vi "PROJE okuma dosya (1).vi"() -> ()   [LabVIEW 2017]
panel:
  out "Waveform Chart":i32[](graph)
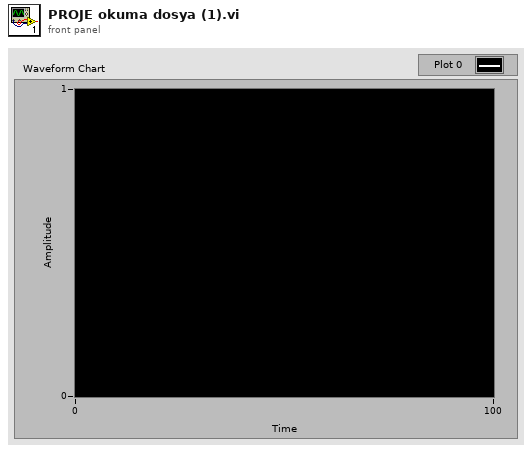
[diagram p1: front panel]
types:
  T1 = enum16{"open", "replace", "create", "open or create", "replace or create", "replace or create with confirmation"}
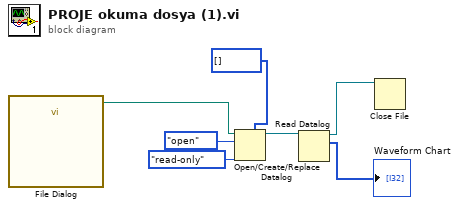
[diagram p0: block diagram]
diagram:
  n1 = call "File Dialog"() -> ("selected path"=w4:path)  [unwired: 12 in, 3 out]
  n2 = Open/Create/Replace Datalog(5:i32[] [], 9:enum16{"read/write", "read-only", "write-only"}."read-only" ("access (0:read/write)"), 10:T1."open" ("operation (0:open)"), 11:w4) -> (3:w3:refnum<k1>)  [unwired: 2 in, 2 out]
  n3 = Read Datalog(7:w3) -> (2:→"Waveform Chart":i32[], 3:w1:refnum<k1>)  [unwired: 2 in, 1 out]
  n4 = Close File(refnum=w1) -> ()  [unwired: 1 in, 2 out]
